vi "SCA-RT_Kubley-timing.vi"() -> ()   [LabVIEW 2016]
uses:
  controls/SCA states.ctl
  Common-Control/Gate Valve Readback.ctl
  controls/Vertical Rod states.ctl
  Common-Control/Horizontal Rod states.ctl
  Common-Control/GP307 cluster.ctl
  controls/SCA commands.ctl
  <vilib>/Platform/TimedLoop/XDataNode/timing_clust.ctl
  <vilib>/Platform/TimedLoop/XDataNode/nitl_modes.ctl
  <vilib>/Platform/TimedLoop/XDataNode/wakeup.ctl
  controls/Encoder bit cluster.ctl
  <vilib>/Analysis/baseanly.llb/Mean (DBL).vi
  <vilib>/Instr/_visa.llb/VISA Configure Serial Port (Instr).vi
  <vilib>/Motion/Express/_s/nimc.fb.straightLineMove.startStraightLineMove.axis.modeRelative.0.vi
  <vilib>/Platform/TimedLoop/XDataNode/loadnilvce.vi
  <vilib>/Motion/BlockNode/FB.NIMotion.xnode
  <vilib>/Platform/TimedLoop/XDataNode/XDataNode.xnode
  <vilib>/Platform/TimedLoop/XDataNode/XDNodeRunTimeDep.lvlib
  <vilib>/Analysis/NI_AALBase.lvlib
  <vilib>/NI_Real-Time Target Support.lvlib
panel:
  out "Immersion Lens I set":dbl
  out "Immersion Lens V Set":dbl
  out "Timeouts Update loop error":errorcluster
  out "SCA Command":T1
  out "Timeouts":T2
  out "Encoder loop error":errorcluster
  out "Convectron readback loop error":errorcluster
  out "HV Control loop error":errorcluster
  out "Rotate Wheel error":errorcluster
  out "Ion Source Vac Cluster":T3
  out "Bellows Vac Cluster":T3
  out "SCA-cRIO error":errorcluster
  in  "Rollover Sample":i8=54
  out "Insert Rod Status":T4
  out "Retract Rod Status":T4
  out "Sample Rod status":T5
  out "Wheel GV":T6
  out "Raw bits":bool[](array[boolean])
  out "Converted bits":bool[](array[boolean])
  out "Immersion Lens I read":dbl format="%0.2f"
  out "Immersion Lens V read":dbl format="%0.2f"
  out "SCA next state":T7
  out "Extractor I read":dbl
  out "Extractor V read":dbl
  out "Extractor V set":dbl
  out "Cathode V read":dbl
  out "Cathode I read":dbl
  out "Cathode V set":dbl
  in  "Execute Move":bool
  out "New Move":dbl
  out "Encoder Destination":dbl
  in  "Step Window Radius":i16=2
  out "In Range?":bool
  out "Window Limit 2":i16
  out "Window Limit 1":i16
  out "Encoder position":u16
  in  "clear error 3":bool
  in  "clear error 2":bool
  in  "clear error":bool
  out "action":string
  out "Vac Readback Loop error":errorcluster
  out "Sample Wheel Convectron":string
  out "Sample Rod UP sensor":bool
  out "Sample Rod DOWN sensor":bool
  out "done":bool
  out "Insert Rod IN sensor":bool
  out "Insert Rod OUT sensor":bool
  out "Retract Rod IN sensor":bool
  out "Retract Rod OUT sensor":bool
  out "Sensor loop error":errorcluster
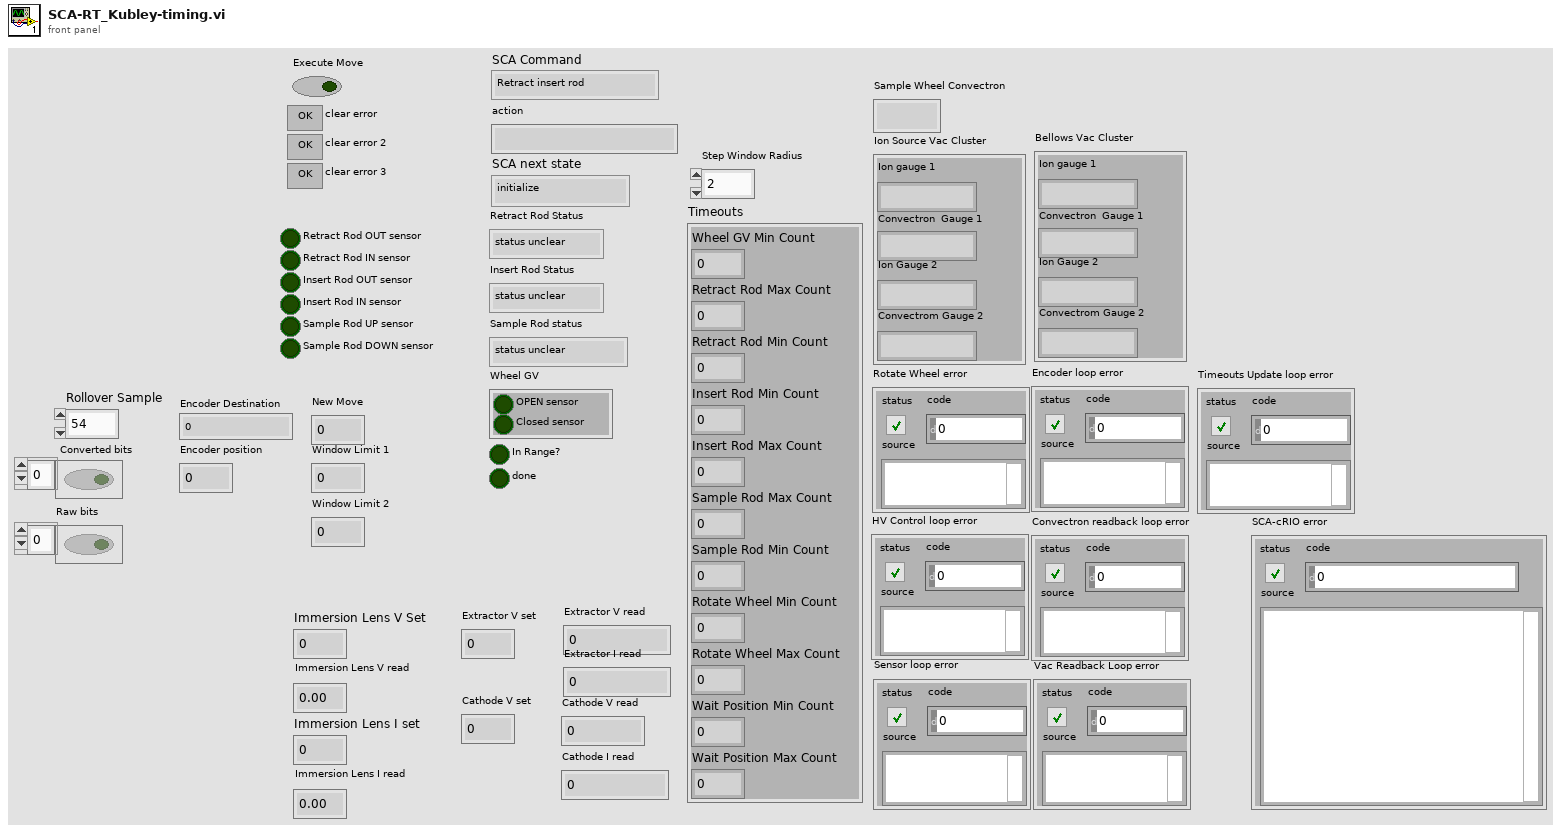
[diagram p1: front panel]
types:
  T1 = typedef "SCA commands.ctl" = enum16{"Retract insert rod", "Insert insert rod", "Retract retract rod", "Insert retract rod", "Retract sample rod", "Insert sample rod", "Open wheel GV", "Close wheel GV", "Open ion source GV", "Close ion source GV", "Pump out source", "Vent source", "Rotate wheel randomly", "Rotate wheel", "Start random sample change", "Start sample change"}
  T2 = cluster{"Wheel GV Min Count":i32, "Retract Rod Max Count":u32, "Retract Rod Min Count":u32, "Insert Rod Min Count":u32, "Insert Rod Max Count":u32, "Sample Rod Max Count":u32, "Sample Rod Min Count":u32, "Rotate Wheel Min Count":u32, "Rotate Wheel Max Count":u32, "Wait Position Min Count":u32, "Wait Position Max Count":u32}
  T3 = typedef "GP307 cluster.ctl" = cluster{"Ion gauge 1":string, "Convectron  Gauge 1 ":string, "Ion Gauge 2":string, "Convectrom Gauge 2":string}
  T4 = typedef "Horizontal Rod states.ctl" = enum16{"status unclear", "rod in", "rod out"}
  T5 = typedef "Vertical Rod states.ctl" = enum16{"status unclear", "rod down", "rod up"}
  T6 = typedef "Gate Valve Readback.ctl" = cluster{"OPEN sensor":bool, "Closed sensor":bool}
  T7 = typedef "SCA states.ctl" = enum16{"initialize", "wait", "change sample start", "change sample", "check position", "wait position", "rotate wheel", "sample change complete", "sample rod up", "sample rod down", "retract rod in", "retract rod out", "insert rod in", "insert rod out", "wheel GV open", "wheel GV close", "vent source", "pump source"}
  T8 = typedef "GV states.ctl" = enum16{"status unclear", "closed", "open"}
  T9 = typedef "XDNodeRunTimeDep.lvlib/timing_clust.ctl" = cluster{"Expected End [f-1]":u64, "Actual End [f-1]":u64, "Finished Late? [f-1]":bool, "Expected End [i-1]":u64, "Actual End [i-1]":u64, "Finished Late? [i-1]":bool, "Expected Start [i]":u64, "Actual Start [i]":u64, "Expected Start [f]":u64, "Actual Start [f]":u64, "Source Name":string, "Structure Name":string, "Period":i64, "Deadline":i64, "Offset":i64, "Start":i64, "Priority":i32, "Timeout":i32, "Mode":T10, "Wakeup Reason":T11, "Error":errorcluster, "Source Type":string, "Secondary Source Type":string, "Global End Time":u64, "Global Start Time":u64, "Frame Duration":u64, "Iteration Duration":u64, "Assigned CPU":i32, "I/O Scan Engine Mode":u32}
  T10 = typedef "XDNodeRunTimeDep.lvlib/nitl_modes.ctl" = enum32{"No Change", "Process missed periods, maintain original phase", "Discard missed periods, maintain original phase", "Process missed periods, ignore original phase", "Discard missed periods, ignore original phase"}
  T11 = typedef "XDNodeRunTimeDep.lvlib/wakeup.ctl" = enum32{"Normal", "Aborted", "Asynchronous wakeup", "Timing source error", "Timed loop error", "Timeout"}
  T12 = typedef "Encoder bit cluster.ctl" = cluster{"MSB":bool, "13th bit":bool, "12th bit":bool, "11th bit":bool, "10th bit":bool, "9th bit":bool, "8th bit":bool, "7th bit":bool, "6th bit":bool, "5th bit":bool, "4th bit":bool, "3rd bit":bool, "2nd bit":bool, "LSB":bool}
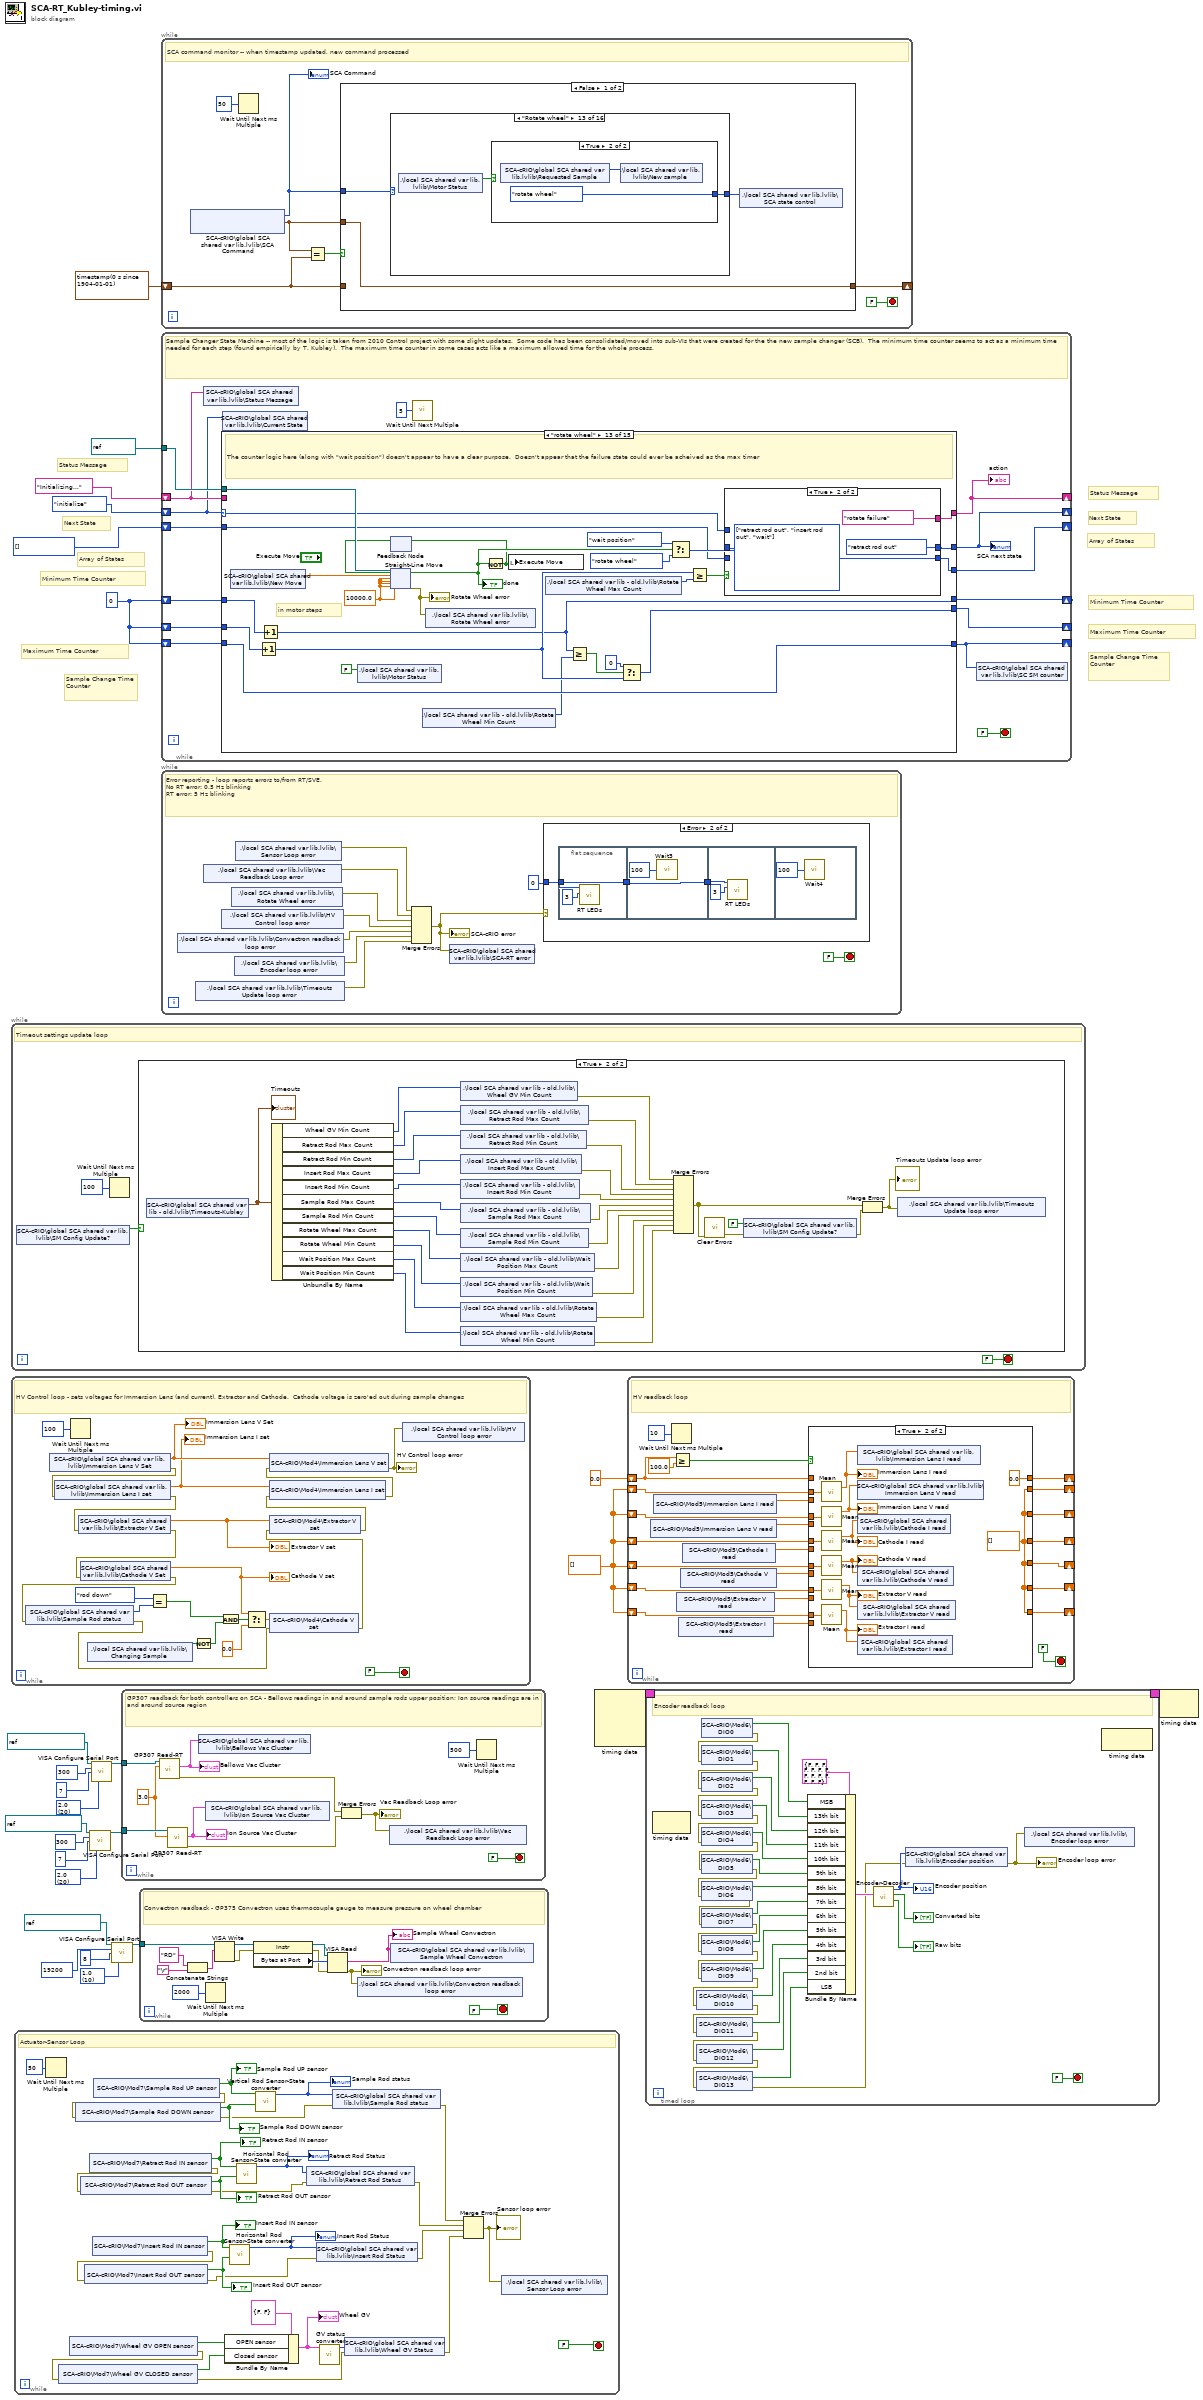
[diagram p0: block diagram]
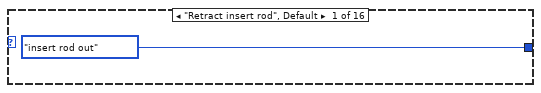
[diagram p2: hidden frame]
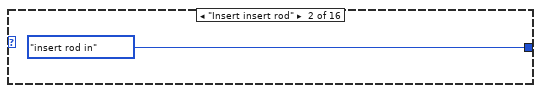
[diagram p3: hidden frame]
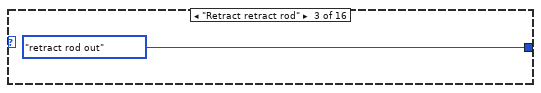
[diagram p4: hidden frame]
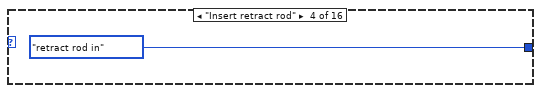
[diagram p5: hidden frame]
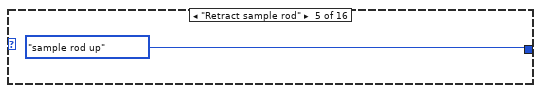
[diagram p6: hidden frame]
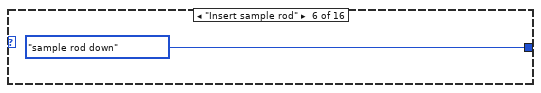
[diagram p7: hidden frame]
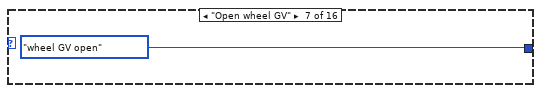
[diagram p8: hidden frame]
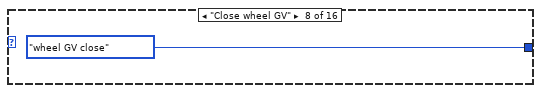
[diagram p9: hidden frame]
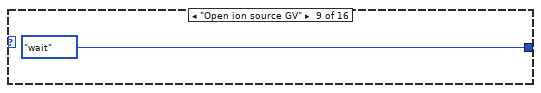
[diagram p10: hidden frame]
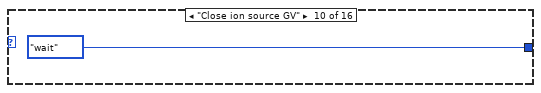
[diagram p11: hidden frame]
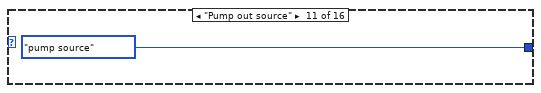
[diagram p12: hidden frame]
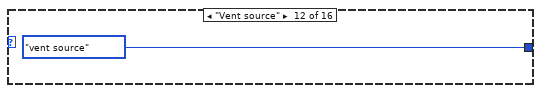
[diagram p13: hidden frame]
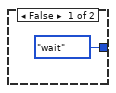
[diagram p14: hidden frame]
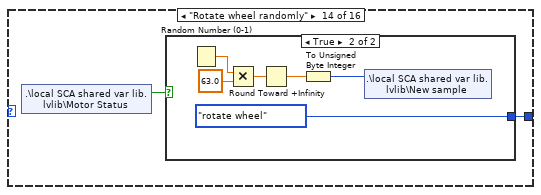
[diagram p15: hidden frame]
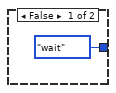
[diagram p16: hidden frame]
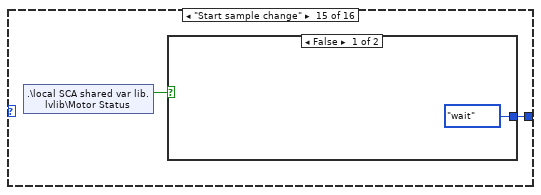
[diagram p17: hidden frame]
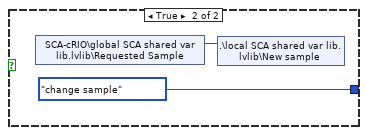
[diagram p18: hidden frame]
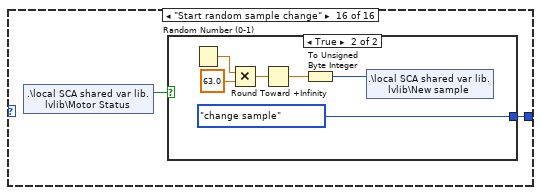
[diagram p19: hidden frame]
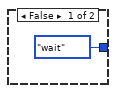
[diagram p20: hidden frame]
diagram:
  w3 = dbl[] []
  w20 = u16 20 items=["1.0"=10, "1.5"=15, "2.0"=20] ("stop bits (10: 1 bit)")
  w24 = u16 10 items=["1.0"=10, "1.5"=15, "2.0"=20] ("stop bits (10: 1 bit)")
  w14 = u16 20 items=["1.0"=10, "1.5"=15, "2.0"=20] ("stop bits (10: 1 bit)")
  w8 = u32 0
  w25 = T7[] [] items=["initialize", "wait", "change sample start", "change sample", "check position", "wait position", "rotate wheel", "sample change complete", "sample rod up", "sample rod down", "retract rod in", "retract rod out", "insert rod in", "insert rod out", "wheel GV open", "wheel GV close", "vent source", "pump source"]
  # "Status Message"
  # "Array of States"
  # "Next State"
  # "Sample Change Time Counter"
  # "Maximum Time Counter"
  # "Minimum Time Counter"
  # "Status Message"
  # "Array of States"
  # "Next State"
  # "Sample Change Time Counter"
  # "Maximum Time Counter"
  # "Minimum Time Counter"
  n1 = while {
    stop <- FALSE stop-if-true
    # "Timeout settings update loop"
    n2 = shared-variable "SCA-cRIO\\global SCA shared var lib.lvlib\\SM Config Update?"() -> (w28:bool)  [unwired: 1 in, 1 out]
    n3 = Wait Until Next ms Multiple(millisecond multiple=u32 100) -> ()  [unwired: 1 out]
    n4 = case shown="True" w28 {
      frame False {
      }
      frame True {
        n5 = shared-variable "SCA-cRIO\\global SCA shared var lib - old.lvlib\\Timeouts-Kubley"() -> (w55:T2)  [unwired: 1 in, 1 out]
        "Timeouts" <- w55
        n6 = Unbundle By Name(w55) -> ("Wheel GV Min Count"=w54:i32, "Retract Rod Max Count"=w53:u32, "Retract Rod Min Count"=w52:u32, "Insert Rod Max Count"=w51:u32, "Insert Rod Min Count"=w50:u32, "Sample Rod Max Count"=w49:u32, "Sample Rod Min Count"=w48:u32, "Rotate Wheel Max Count"=w47:u32, "Rotate Wheel Min Count"=w46:u32, "Wait Position Max Count"=w45:u32, "Wait Position Min Count"=w44:u32)
        n7 = shared-variable ".\\local SCA shared var lib - old.lvlib\\Wheel GV Min Count"(w54) -> (error out=w43:errorcluster)  [unwired: 1 in]
        n8 = shared-variable ".\\local SCA shared var lib - old.lvlib\\Retract Rod Max Count"(w53) -> (error out=w42:errorcluster)  [unwired: 1 in]
        n9 = shared-variable ".\\local SCA shared var lib - old.lvlib\\Retract Rod Min Count"(w52) -> (error out=w41:errorcluster)  [unwired: 1 in]
        n10 = shared-variable ".\\local SCA shared var lib - old.lvlib\\Insert Rod Max Count"(w51) -> (error out=w40:errorcluster)  [unwired: 1 in]
        n11 = shared-variable ".\\local SCA shared var lib - old.lvlib\\Insert Rod Min Count"(w50) -> (error out=w39:errorcluster)  [unwired: 1 in]
        n12 = shared-variable ".\\local SCA shared var lib - old.lvlib\\Sample Rod Max Count"(w49) -> (error out=w38:errorcluster)  [unwired: 1 in]
        n13 = shared-variable ".\\local SCA shared var lib - old.lvlib\\Sample Rod Min Count"(w48) -> (error out=w37:errorcluster)  [unwired: 1 in]
        n14 = shared-variable ".\\local SCA shared var lib - old.lvlib\\Wait Position Max Count"(w47) -> (error out=w36:errorcluster)  [unwired: 1 in]
        n15 = shared-variable ".\\local SCA shared var lib - old.lvlib\\Wait Position Min Count"(w46) -> (error out=w35:errorcluster)  [unwired: 1 in]
        n16 = shared-variable ".\\local SCA shared var lib - old.lvlib\\Rotate Wheel Max Count"(w45) -> (error out=w34:errorcluster)  [unwired: 1 in]
        n17 = shared-variable ".\\local SCA shared var lib - old.lvlib\\Rotate Wheel Min Count"(w44) -> (error out=w33:errorcluster)  [unwired: 1 in]
        n18 = Merge Errors(w43, w42, w41, w40, w39, w38, w37, w36, w35, w34, w33) -> (w31:errorcluster)
        n19 = call <vilib>:"Clear Errors.vi"("error in (no error)"=w31) -> ("error out"=w32:errorcluster)  [unwired: 5 in, 1 out]
        n20 = shared-variable "SCA-cRIO\\global SCA shared var lib.lvlib\\SM Config Update?"(FALSE ("SM Config Update?"), error in=w32) -> (error out=w30:errorcluster)
        n21 = Merge Errors(w31, w30) -> (w29:errorcluster)
        "Timeouts Update loop error" <- w29
        n22 = shared-variable ".\\local SCA shared var lib.lvlib\\Timeouts Update loop error"(w29) -> ()  [unwired: 1 in, 1 out]
      }
    }
  }
  n23 = while {
    stop <- FALSE stop-if-true
    # "HV Control loop - sets voltages for Immersion Lens (and current), Extractor and Cathode.  Cathode voltage is zero'ed out during sample changes"
    n24 = shared-variable "SCA-cRIO\\global SCA shared var lib.lvlib\\Immersion Lens V Set"() -> (w71:dbl, error out=w69:errorcluster)  [unwired: 1 in]
    "Immersion Lens V Set" <- w71
    n25 = shared-variable "SCA-cRIO\\global SCA shared var lib.lvlib\\Immersion Lens I set"(error in=w69) -> (w70:dbl, error out=w68:errorcluster)
    "Immersion Lens I set" <- w70
    n26 = Wait Until Next ms Multiple(millisecond multiple=u32 100) -> ()  [unwired: 1 out]
    n27 = shared-variable "SCA-cRIO\\global SCA shared var lib.lvlib\\Extractor V Set"(error in=w68) -> (w77:dbl, error out=w67:errorcluster)
    "Extractor V set" <- w77
    n28 = shared-variable "SCA-cRIO\\global SCA shared var lib.lvlib\\Cathode V Set"(error in=w67) -> (w74:dbl, error out=w66:errorcluster)
    "Cathode V set" <- w74
    n29 = shared-variable "SCA-cRIO\\global SCA shared var lib.lvlib\\Sample Rod status"(error in=w66) -> (w60:T5, error out=w58:errorcluster)
    n30 = shared-variable ".\\local SCA shared var lib.lvlib\\Changing Sample"() -> (w76:bool)  [unwired: 1 in, 1 out]
    n31 = Equal?(x=Vertical_Rod_states."rod down", y=w60) -> (x = y?=w61:bool)
    n32 = Not(x=w76) -> (.not. x?=w57:bool)
    n33 = And(x=w61, y=w57) -> (x .and. y?=w75:bool)
    n34 = Select(t=w74, s=w75, f=0.0) -> (s? t:f=w72:dbl)
    n35 = shared-variable "SCA-cRIO\\Mod4\\Cathode V set"(w72, error in=w58) -> (error out=w63:errorcluster)
    n36 = shared-variable "SCA-cRIO\\Mod4\\Extractor V set"(w77, error in=w63) -> (error out=w64:errorcluster)
    n37 = shared-variable "SCA-cRIO\\Mod4\\Immersion Lens I set"(w70, error in=w64) -> (error out=w65:errorcluster)
    n38 = shared-variable "SCA-cRIO\\Mod4\\Immersion Lens V set"(w71, error in=w65) -> (error out=w62:errorcluster)
    "HV Control loop error" <- w62
    n39 = shared-variable ".\\local SCA shared var lib.lvlib\\HV Control loop error"(w62) -> ()  [unwired: 1 in, 1 out]
  }
  n40 = while {
    stop <- FALSE ("stop") stop-if-true
    # "Actuator-Sensor Loop"
    n41 = Wait Until Next ms Multiple(millisecond multiple=u32 50) -> ()  [unwired: 1 out]
    n42 = shared-variable "SCA-cRIO\\Mod7\\Wheel GV OPEN sensor"() -> (w103:bool, error out=w89:errorcluster)  [unwired: 1 in]
    n43 = shared-variable "SCA-cRIO\\Mod7\\Wheel GV CLOSED sensor"(error in=w89) -> (w104:bool, error out=w88:errorcluster)
    n44 = shared-variable "SCA-cRIO\\Mod7\\Retract Rod IN sensor"() -> (w98:bool, error out=w91:errorcluster)  [unwired: 1 in]
    "Retract Rod IN sensor" <- w98
    n45 = shared-variable "SCA-cRIO\\Mod7\\Retract Rod OUT sensor"(error in=w91) -> (w97:bool, error out=w85:errorcluster)
    "Retract Rod OUT sensor" <- w97
    n46 = shared-variable "SCA-cRIO\\Mod7\\Insert Rod IN sensor"() -> (w96:bool, error out=w90:errorcluster)  [unwired: 1 in]
    "Insert Rod IN sensor" <- w96
    n47 = shared-variable "SCA-cRIO\\Mod7\\Insert Rod OUT sensor"(error in=w90) -> (w95:bool, error out=w87:errorcluster)
    "Insert Rod OUT sensor" <- w95
    n48 = shared-variable "SCA-cRIO\\Mod7\\Sample Rod UP sensor"() -> (w101:bool, error out=w92:errorcluster)  [unwired: 1 in]
    "Sample Rod UP sensor" <- w101
    n49 = shared-variable "SCA-cRIO\\Mod7\\Sample Rod DOWN sensor"(error in=w92) -> (w100:bool, error out=w86:errorcluster)
    "Sample Rod DOWN sensor" <- w100
    n50 = Bundle By Name(cluster=T6 {"OPEN sensor"=FALSE, "Closed sensor"=FALSE} ("Gate Valve"), "OPEN sensor"=w103, "Closed sensor"=w104) -> (w106:T6)
    "Wheel GV" <- w106
    n51 = call "Horizontal Rod Sensor-State converter.vi"("IN Sensor"=w96, "OUT Sensor"=w95) -> ("Status"=w94:T4)  [unwired: 8 in]
    "Insert Rod Status" <- w94
    n52 = call "Horizontal Rod Sensor-State converter.vi"("IN Sensor"=w98, "OUT Sensor"=w97) -> ("Status"=w93:T4)  [unwired: 8 in]
    "Retract Rod Status" <- w93
    n53 = call "Vertical Rod Sensor-State converter.vi"("UP Sensor"=w101, "DOWN Sensor"=w100) -> ("Status"=w99:T5)  [unwired: 8 in]
    "Sample Rod status" <- w99
    n54 = shared-variable "SCA-cRIO\\global SCA shared var lib.lvlib\\Retract Rod Status"(w93, error in=w85) -> (error out=w82:errorcluster)
    n55 = shared-variable "SCA-cRIO\\global SCA shared var lib.lvlib\\Insert Rod Status"(w94, error in=w87) -> (error out=w81:errorcluster)
    n56 = call "GV status converter.vi"("Gate Valve"=w106) -> ("GV Status"=w102:T8)  [unwired: 10 in]
    n57 = shared-variable "SCA-cRIO\\global SCA shared var lib.lvlib\\Sample Rod status"(w99, error in=w86) -> (error out=w83:errorcluster)
    n58 = shared-variable "SCA-cRIO\\global SCA shared var lib.lvlib\\Wheel GV Status"(w102, error in=w88) -> (error out=w80:errorcluster)
    n59 = Merge Errors(w83, w82, w81, w80) -> (w84:errorcluster)
    "Sensor loop error" <- w84
    n60 = shared-variable ".\\local SCA shared var lib.lvlib\\Sensor Loop error"(w84) -> ()  [unwired: 1 in, 1 out]
  }
  n61 = call-poly "VISA Configure Serial Port"("VISA resource name"=refnum<visa-resource-name> "ASRL6::INSTR", "baud rate (9600)"=u32 300, "data bits (8)"=u16 7, "stop bits (10: 1 bit)"=w14) -> ("VISA resource name out"=w15:refnum<visa-resource-name>)  [unwired: 10 in, 1 out]
  n62 = call-poly "VISA Configure Serial Port"("VISA resource name"=refnum<visa-resource-name> "ASRL8::INSTR", "baud rate (9600)"=u32 300, "data bits (8)"=u16 7, "stop bits (10: 1 bit)"=w20) -> ("VISA resource name out"=w21:refnum<visa-resource-name>)  [unwired: 10 in, 1 out]
  n63 = call-poly "VISA Configure Serial Port"("VISA resource name"=refnum<visa-resource-name> "ASRL7::INSTR", "baud rate (9600)"=u32 19200, "data bits (8)"=u16 8, "stop bits (10: 1 bit)"=w24) -> ("VISA resource name out"=w10:refnum<visa-resource-name>)  [unwired: 10 in, 1 out]
  n64 = while {
    tunnel: w15 -> [w112]
    tunnel: w21 -> [w115]
    stop <- FALSE ("stop 4") stop-if-true
    w111 = 3.0 ("Delay Time (s)")
    # "GP307 readback for both controllers on SCA - Bellows readings in and around sample rods upper position; Ion source readings are in and around source region"
    n65 = call "GP307 Read-RT.vi"("Delay Time (s)"=w111, "VISA Refnum in"=w115) -> ("error out"=w113:errorcluster, "GP307 output"=w114:T3)  [unwired: 7 in, 1 out]
    "Bellows Vac Cluster" <- w114
    n66 = call "GP307 Read-RT.vi"("Delay Time (s)"=w111, "VISA Refnum in"=w112) -> ("error out"=w109:errorcluster, "GP307 output"=w110:T3)  [unwired: 7 in, 1 out]
    "Ion Source Vac Cluster" <- w110
    n67 = shared-variable "SCA-cRIO\\global SCA shared var lib.lvlib\\Bellows Vac Cluster"(w114) -> ()  [unwired: 1 in, 1 out]
    n68 = shared-variable "SCA-cRIO\\global SCA shared var lib.lvlib\\Ion Source Vac Cluster"(w110) -> ()  [unwired: 1 in, 1 out]
    n69 = Merge Errors(w113, w109) -> (w116:errorcluster)
    "Vac Readback Loop error" <- w116
    n70 = shared-variable ".\\local SCA shared var lib.lvlib\\Vac Readback Loop error"(w116) -> ()  [unwired: 1 in, 1 out]
    n71 = Wait Until Next ms Multiple(millisecond multiple=u32 500) -> ()  [unwired: 1 out]
  }
  n72 = while {
    tunnel: w10 -> [w124]
    stop <- FALSE ("stop 3") stop-if-true
    # "Convectron readback - GP375 Convectron uses thermocouple gauge to measure pressure on wheel chamber"
    n73 = Concatenate Strings("RD" ("write buffer 2"), "\r") -> (w131:string)
    n74 = Wait Until Next ms Multiple(millisecond multiple=u32 2000) -> ()  [unwired: 1 out]
    n75 = VISA Write(VISA resource name=w124, write buffer=w131) -> (VISA resource name out=w125:refnum<visa-resource-name>, error out=w121:errorcluster)  [unwired: 1 in, 1 out]
    n76 = property class="Instr"(reference=w125, error in=w121) -> (reference out=w126:refnum<visa-resource-name>, error out=w120:errorcluster, "Bytes at Port"=w127:u32)
    n77 = VISA Read(VISA resource name=w126, byte count=w127, error in (no error)=w120) -> (read buffer=w122:string, error out=w119:errorcluster)  [unwired: 2 out]
    "Sample Wheel Convectron" <- w122
    "Convectron readback loop error" <- w119
    n78 = shared-variable ".\\local SCA shared var lib.lvlib\\Convectron readback loop error"(w119) -> ()  [unwired: 1 in, 1 out]
    n79 = shared-variable "SCA-cRIO\\global SCA shared var lib.lvlib\\Sample Wheel Convectron"(w122) -> ()  [unwired: 1 in, 1 out]
  }
  n80 = while {
    shift-right: [w144] -> _
    shift-left: SCA_states."initialize" ("SC2 state") -> [w134]
    shift-right: [w133] -> _
    shift-left: w25 -> [w143]
    shift-right: [w141] -> _
    shift-left: w8 -> [w142]
    shift-right: [w140] -> _
    shift-left: "Initializing..." -> [w135]
    shift-right: [w138] -> _
    shift-left: w8 -> [w139]
    shift-right: [w136] -> _
    shift-left: w8 -> [w137]
    tunnel: refnum<k21> "Axis 1" ("resource") -> [w145]
    stop <- FALSE ("stop 2") stop-if-true
    # "Sample Changer State Machine -- most of the logic is taken from 2010 Control project with some slight updates.  Some code has been consolidated/moved into sub-VIs that were created for the the new sample changer (SCB).  The minimum time counter seems to act as a minimum time needed for each step (found empirically by T. Kubley).  The maximum time counter in some cases acts like a maximum allowed time for the whole process."
    n81 = shared-variable "SCA-cRIO\\global SCA shared var lib.lvlib\\Status Message"(w135) -> ()  [unwired: 1 in, 1 out]
    n82 = case shown="\"rotate wheel\"" w134 {
      selector: w134 -> [_ _ _ _ w219 w237 w260 w294 w328 w362 w396 w430 w466 w521 w551]
      tunnel: w145 -> [_ _ _ _ _ _ _ _ _ _ _ _ w481 _ _]
      tunnel: [SCA_states."wait" ("SC2 state") w170 w200 w210 w224 w243 w268 w302 w336 w370 w404 w438 w475 w522 w561] -> w144
      tunnel: w143 -> [w160 _ w192 w202 w220 w238 w261 w295 w329 w363 w397 w431 w467 w520 w550]
      tunnel: w142 -> [w163 _ _ _ w227 w246 w274 w308 w342 w376 w410 w444 w479 w532 w556]
      tunnel: [w163 w173 w195 w205 w226 w245 w254 w288 w323 w357 w391 w425 w462 w533 w556] -> w141
      tunnel: [w160 w171 w192 w202 w220 w238 w263 w297 w331 w365 w399 w433 w476 w529 w550] -> w133
      tunnel: w135 -> [w161 w176 w198 w208 _ _ _ _ _ _ _ _ _ _ _]
      tunnel: [w161 w175 w197 w207 w223 w242 w270 w304 w338 w372 w406 w440 w474 w528 w560] -> w140
      tunnel: w139 -> [w164 _ _ _ w225 w244 w267 w301 w335 w369 w403 w437 w477 w530 _]
      tunnel: [w164 w173 w195 w205 w212 w241 w265 w299 w333 w367 w401 w435 w470 w524 u32 0 ("t")] -> w138
      tunnel: w137 -> [w165 _ _ _ w222 w240 w264 w298 w332 w366 w400 w434 w461 w517 w559]
      tunnel: [w165 w173 w195 w205 w222 w240 w264 w298 w332 w366 w400 w434 w461 w517 w559] -> w136
      frame "initialize" {
        n83 = shared-variable ".\\local SCA shared var lib.lvlib\\Motor Status"(TRUE ("Motor Status")) -> ()  [unwired: 1 in, 1 out]
        n84 = shared-variable ".\\local SCA shared var lib.lvlib\\Changing Sample"(FALSE ("Changing Sample")) -> ()  [unwired: 1 in, 1 out]
        n85 = shared-variable "SCA-cRIO\\global SCA shared var lib - old.lvlib\\Start Sample Change"(FALSE ("start sample change")) -> (error out=w168:errorcluster)  [unwired: 1 in]
        n86 = shared-variable ".\\local SCA shared var lib - old.lvlib\\Rotate Wheel Max Count"(u32 800 ("Rotate Wheel Max Count")) -> ()  [unwired: 1 in, 1 out]
        n87 = shared-variable ".\\local SCA shared var lib - old.lvlib\\Wait Position Min Count"(u32 8000 ("y")) -> ()  [unwired: 1 in, 1 out]
        n88 = shared-variable ".\\local SCA shared var lib - old.lvlib\\Wait Position Max Count"(u32 1500 ("y")) -> ()  [unwired: 1 in, 1 out]
        n89 = shared-variable ".\\local SCA shared var lib - old.lvlib\\Rotate Wheel Min Count"(u32 350 ("Rotate Wheel Min Count")) -> ()  [unwired: 1 in, 1 out]
        n90 = shared-variable "SCA-cRIO\\global SCA shared var lib - old.lvlib\\change sample start end"(FALSE ("change sample start end"), error in=w168) -> ()  [unwired: 1 out]
        n91 = shared-variable ".\\local SCA shared var lib - old.lvlib\\Insert Rod Min Count"(u32 30 ("y")) -> ()  [unwired: 1 in, 1 out]
        n92 = shared-variable ".\\local SCA shared var lib - old.lvlib\\Insert Rod Max Count"(u32 500 ("y")) -> ()  [unwired: 1 in, 1 out]
        n93 = shared-variable ".\\local SCA shared var lib - old.lvlib\\Wheel GV Min Count"(70 ("Wheel GV Min Time")) -> ()  [unwired: 1 in, 1 out]
        n94 = shared-variable ".\\local SCA shared var lib - old.lvlib\\Sample Rod Min Count"(u32 10 ("y")) -> ()  [unwired: 1 in, 1 out]
        n95 = shared-variable ".\\local SCA shared var lib - old.lvlib\\Sample Rod Max Count"(u32 1000 ("y")) -> ()  [unwired: 1 in, 1 out]
        n96 = shared-variable ".\\local SCA shared var lib - old.lvlib\\Retract Rod Max Count"(u32 200 ("y")) -> ()  [unwired: 1 in, 1 out]
        n97 = shared-variable ".\\local SCA shared var lib - old.lvlib\\Retract Rod Min Count"(u32 30 ("y")) -> ()  [unwired: 1 in, 1 out]
      }
      frame "wait", Default {
        w173 = u32 0
        n98 = shared-variable ".\\local SCA shared var lib.lvlib\\SCA state control"() -> (w169:T7)  [unwired: 1 in, 1 out]
        n99 = case shown="\"change sample\"" w169 {
          tunnel: [w178 w179 w180 w181 w182 w183 w184 w185 w186 w187 w188 w189 w190] -> w171
          frame "wheel GV close" {
            w178 = T7[] [enum."wheel GV close", enum."wait"] items=["initialize", "wait", "change sample start", "change sample", "check position", "wait position", "rotate wheel", "sample change complete", "sample rod up", "sample rod down", "retract rod in", "retract rod out", "insert rod in", "insert rod out", "wheel GV open", "wheel GV close", "vent source", "pump source"]
          }
          frame "wheel GV open" {
            w179 = T7[] [enum."wheel GV open", enum."wait"] items=["initialize", "wait", "change sample start", "change sample", "check position", "wait position", "rotate wheel", "sample change complete", "sample rod up", "sample rod down", "retract rod in", "retract rod out", "insert rod in", "insert rod out", "wheel GV open", "wheel GV close", "vent source", "pump source"]
          }
          frame "sample rod up" {
            w180 = T7[] [enum."sample rod up", enum."wait"] items=["initialize", "wait", "change sample start", "change sample", "check position", "wait position", "rotate wheel", "sample change complete", "sample rod up", "sample rod down", "retract rod in", "retract rod out", "insert rod in", "insert rod out", "wheel GV open", "wheel GV close", "vent source", "pump source"]
          }
          frame "sample rod down" {
            w181 = T7[] [enum."sample rod down", enum."wait"] items=["initialize", "wait", "change sample start", "change sample", "check position", "wait position", "rotate wheel", "sample change complete", "sample rod up", "sample rod down", "retract rod in", "retract rod out", "insert rod in", "insert rod out", "wheel GV open", "wheel GV close", "vent source", "pump source"]
          }
          frame "retract rod in" {
            w182 = T7[] [enum."retract rod in", enum."wait"] items=["initialize", "wait", "change sample start", "change sample", "check position", "wait position", "rotate wheel", "sample change complete", "sample rod up", "sample rod down", "retract rod in", "retract rod out", "insert rod in", "insert rod out", "wheel GV open", "wheel GV close", "vent source", "pump source"]
          }
          frame "retract rod out" {
            w183 = T7[] [enum."retract rod out", enum."wait"] items=["initialize", "wait", "change sample start", "change sample", "check position", "wait position", "rotate wheel", "sample change complete", "sample rod up", "sample rod down", "retract rod in", "retract rod out", "insert rod in", "insert rod out", "wheel GV open", "wheel GV close", "vent source", "pump source"]
          }
          frame "insert rod in" {
            w184 = T7[] [enum."insert rod in", enum."wait"] items=["initialize", "wait", "change sample start", "change sample", "check position", "wait position", "rotate wheel", "sample change complete", "sample rod up", "sample rod down", "retract rod in", "retract rod out", "insert rod in", "insert rod out", "wheel GV open", "wheel GV close", "vent source", "pump source"]
          }
          frame "insert rod out" {
            w185 = T7[] [enum."insert rod out", enum."wait"] items=["initialize", "wait", "change sample start", "change sample", "check position", "wait position", "rotate wheel", "sample change complete", "sample rod up", "sample rod down", "retract rod in", "retract rod out", "insert rod in", "insert rod out", "wheel GV open", "wheel GV close", "vent source", "pump source"]
          }
          frame "rotate wheel" {
            w186 = T7[] [enum."check position", enum."wait"] items=["initialize", "wait", "change sample start", "change sample", "check position", "wait position", "rotate wheel", "sample change complete", "sample rod up", "sample rod down", "retract rod in", "retract rod out", "insert rod in", "insert rod out", "wheel GV open", "wheel GV close", "vent source", "pump source"]
          }
          frame "change sample" {
            w187 = T7[] [enum."change sample start", enum."sample rod up", enum."retract rod in", enum."retract rod out", enum."check position", enum."insert rod in", enum."insert rod out", enum."sample rod down", enum."sample change complete", enum."wait"] items=["initialize", "wait", "change sample start", "change sample", "check position", "wait position", "rotate wheel", "sample change complete", "sample rod up", "sample rod down", "retract rod in", "retract rod out", "insert rod in", "insert rod out", "wheel GV open", "wheel GV close", "vent source", "pump source"]
          }
          frame "vent source" {
            w188 = T7[] [enum."sample rod up", enum."retract rod in", enum."retract rod out", enum."insert rod out", enum."wheel GV close", enum."wait"] items=["initialize", "wait", "change sample start", "change sample", "check position", "wait position", "rotate wheel", "sample change complete", "sample rod up", "sample rod down", "retract rod in", "retract rod out", "insert rod in", "insert rod out", "wheel GV open", "wheel GV close", "vent source", "pump source"]
          }
          frame "pump source" {
            w189 = T7[] [enum."wheel GV open", enum."sample rod up", enum."check position", enum."insert rod in", enum."insert rod out", enum."sample rod down", enum."wait"] items=["initialize", "wait", "change sample start", "change sample", "check position", "wait position", "rotate wheel", "sample change complete", "sample rod up", "sample rod down", "retract rod in", "retract rod out", "insert rod in", "insert rod out", "wheel GV open", "wheel GV close", "vent source", "pump source"]
          }
          frame "wait", Default {
            w190 = T7[] [enum."wait"] items=["initialize", "wait", "change sample start", "change sample", "check position", "wait position", "rotate wheel", "sample change complete", "sample rod up", "sample rod down", "retract rod in", "retract rod out", "insert rod in", "insert rod out", "wheel GV open", "wheel GV close", "vent source", "pump source"]
          }
        }
        n100 = Select(t="Ready", s="clear error", f=w176) -> (s? t:f=w175:string)
        n101 = Index Array(array=w171, index=0) -> (element=w170:T7)
      }
      frame "change sample start" {
        w195 = u32 0
        n102 = Index Array(array=w192, index=1) -> (element=w200:T7)
        n103 = shared-variable "SCA-cRIO\\global SCA shared var lib - old.lvlib\\change sample start end"(FALSE ("change sample start end")) -> ()  [unwired: 1 in, 1 out]
        n104 = shared-variable ".\\local SCA shared var lib.lvlib\\Changing Sample"(TRUE ("Changing Sample")) -> ()  [unwired: 1 in, 1 out]
        n105 = Select(t="Ready", s="clear error 2", f=w198) -> (s? t:f=w197:string)
      }
      frame "sample change complete" {
        w205 = u32 0
        n106 = shared-variable "SCA-cRIO\\global SCA shared var lib - old.lvlib\\change sample start end"(TRUE ("change sample start end")) -> ()  [unwired: 1 in, 1 out]
        n107 = shared-variable ".\\local SCA shared var lib.lvlib\\Changing Sample"(FALSE ("Changing Sample")) -> ()  [unwired: 1 in, 1 out]
        n108 = Array Size(array=w202) -> (size(s)=w203:i32)
        n109 = Index Array(array=w202, index=w203) -> (element=w210:T7)
        n110 = Select(t="Ready", s="clear error 3", f=w208) -> (s? t:f=w207:string)
      }
      frame "wheel GV open" {
        n111 = call "Modify array of SCA states.vi"("Current State"=w219, "Array of states to process"=w220) -> ("Next State"=w221:T7)  [unwired: 7 in, 1 out]
        n112 = shared-variable "SCA-cRIO\\Mod8\\Wheel GV Actuator"(TRUE ("sc gate valve")) -> (error out=w217:errorcluster)  [unwired: 1 in]
        n113 = shared-variable "SCA-cRIO\\global SCA shared var lib.lvlib\\Wheel GV Status"(error in=w217) -> (w216:enum16{"status unclear", "closed", "open"})  [unwired: 1 out]
        n114 = shared-variable ".\\local SCA shared var lib - old.lvlib\\Wheel GV Min Count"() -> (w211:i32)  [unwired: 1 in, 1 out]
        n115 = Equal?(x=enum16{"status unclear", "closed", "open"}."open", y=w216) -> (x = y?=w214:bool)
        n116 = Select(t=w227, s=w214, f=u32 0) -> (s? t:f=w230:u32)
        n117 = Increment(x=w230) -> (x+1=w226:u32)
        n118 = Greater Or Equal?(x=w226, y=w211) -> (x >= y?=w228:bool)
        n119 = Select(t=w221, s=w228, f=w219) -> (s? t:f=w224:T7)
        n120 = Increment(x=w225) -> (x+1=w212:u32)
        n121 = Format Into String(format string="%s", w219) -> (resulting string=w223:string)  [unwired: 2 in, 1 out]
      }
      frame "wheel GV close" {
        n122 = call "Modify array of SCA states.vi"("Current State"=w237, "Array of states to process"=w238) -> ("Next State"=w239:T7)  [unwired: 7 in, 1 out]
        n123 = shared-variable "SCA-cRIO\\Mod8\\Wheel GV Actuator"(FALSE ("sc gate valve")) -> (error out=w235:errorcluster)  [unwired: 1 in]
        n124 = shared-variable "SCA-cRIO\\global SCA shared var lib.lvlib\\Wheel GV Status"(error in=w235) -> (w234:enum16{"status unclear", "closed", "open"})  [unwired: 1 out]
        n125 = shared-variable ".\\local SCA shared var lib - old.lvlib\\Wheel GV Min Count"() -> (w250:i32)  [unwired: 1 in, 1 out]
        n126 = Equal?(x=enum16{"status unclear", "closed", "open"}."closed", y=w234) -> (x = y?=w232:bool)
        n127 = Select(t=w246, s=w232, f=u32 0) -> (s? t:f=w249:u32)
        n128 = Increment(x=w249) -> (x+1=w245:u32)
        n129 = Greater Or Equal?(x=w245, y=w250) -> (x >= y?=w247:bool)
        n130 = Select(t=w239, s=w247, f=w237) -> (s? t:f=w243:T7)
        n131 = Increment(x=w244) -> (x+1=w241:u32)
        n132 = Format Into String(format string="%s", w237) -> (resulting string=w242:string)  [unwired: 2 in, 1 out]
      }
      frame "sample rod up" {
        n133 = Increment(x=w267) -> (x+1=w253:u32)
        n134 = shared-variable "SCA-cRIO\\Mod8\\Sample Rod Actuator"(FALSE ("Sample Rod Actuator")) -> (error out=w258:errorcluster)  [unwired: 1 in]
        n135 = shared-variable ".\\local SCA shared var lib - old.lvlib\\Sample Rod Max Count"() -> (w252:u32)  [unwired: 1 in, 1 out]
        n136 = call "Modify array of SCA states.vi"("Current State"=w260, "Array of states to process"=w261) -> ("Next State"=w262:T7)  [unwired: 7 in, 1 out]
        n137 = shared-variable "SCA-cRIO\\global SCA shared var lib.lvlib\\Sample Rod status"(error in=w258) -> (w257:T5)  [unwired: 1 out]
        n138 = Greater Or Equal?(x=w253, y=w252) -> (x >= y?=w266:bool)
        n139 = shared-variable ".\\local SCA shared var lib - old.lvlib\\Sample Rod Min Count"() -> (w251:u32)  [unwired: 1 in, 1 out]
        n140 = Equal?(x=w257, y=Vertical_Rod_states."rod up") -> (x = y?=w255:bool)
        n141 = Select(t=w274, s=w255, f=u32 0) -> (s? t:f=w272:u32)
        n142 = Increment(x=w272) -> (x+1=w254:u32)
        n143 = Greater Or Equal?(x=w254, y=w251) -> (x >= y?=w273:bool)
        n144 = Select(t=w262, s=w273, f=w260) -> (s? t:f=w269:T7)
        n145 = case shown="False" w266 {
          tunnel: [w280 u32 0] -> w265
          tunnel: [w278 w281] -> w263
          tunnel: [w279 SCA_states."wait" ("SC2 state")] -> w268
          tunnel: w253 -> [w280 _]
          tunnel: w260 -> [w276 _]
          tunnel: [w275 "sample rod failure"] -> w270
          tunnel: w269 -> [w279 _]
          tunnel: w261 -> [w278 _]
          frame False {
            n146 = Format Into String(format string="%s", w276) -> (resulting string=w275:string)  [unwired: 2 in, 1 out]
          }
          frame True {
            w281 = T7[] [enum."wait", enum."insert rod out", enum."wait"] items=["initialize", "wait", "change sample start", "change sample", "check position", "wait position", "rotate wheel", "sample change complete", "sample rod up", "sample rod down", "retract rod in", "retract rod out", "insert rod in", "insert rod out", "wheel GV open", "wheel GV close", "vent source", "pump source"]
          }
        }
      }
      frame "sample rod down" {
        n147 = Increment(x=w301) -> (x+1=w287:u32)
        n148 = shared-variable "SCA-cRIO\\Mod8\\Sample Rod Actuator"(TRUE ("Sample Rod Actuator")) -> (error out=w292:errorcluster)  [unwired: 1 in]
        n149 = shared-variable ".\\local SCA shared var lib - old.lvlib\\Sample Rod Max Count"() -> (w285:u32)  [unwired: 1 in, 1 out]
        n150 = call "Modify array of SCA states.vi"("Current State"=w294, "Array of states to process"=w295) -> ("Next State"=w296:T7)  [unwired: 7 in, 1 out]
        n151 = shared-variable "SCA-cRIO\\global SCA shared var lib.lvlib\\Sample Rod status"(error in=w292) -> (w291:T5)  [unwired: 1 out]
        n152 = Greater Or Equal?(x=w287, y=w285) -> (x >= y?=w300:bool)
        n153 = shared-variable ".\\local SCA shared var lib - old.lvlib\\Sample Rod Min Count"() -> (w286:u32)  [unwired: 1 in, 1 out]
        n154 = Equal?(x=w291, y=Vertical_Rod_states."rod down") -> (x = y?=w289:bool)
        n155 = Select(t=w308, s=w289, f=u32 0) -> (s? t:f=w306:u32)
        n156 = Increment(x=w306) -> (x+1=w288:u32)
        n157 = Greater Or Equal?(x=w288, y=w286) -> (x >= y?=w307:bool)
        n158 = Select(t=w296, s=w307, f=w294) -> (s? t:f=w303:T7)
        n159 = case shown="True" w300 {
          tunnel: [w314 u32 0] -> w299
          tunnel: [w312 w315] -> w297
          tunnel: [w313 SCA_states."wait" ("SC2 state")] -> w302
          tunnel: w287 -> [w314 _]
          tunnel: w294 -> [w310 _]
          tunnel: [w309 "sample rod failure"] -> w304
          tunnel: w303 -> [w313 _]
          tunnel: w295 -> [w312 _]
          frame False {
            n160 = Format Into String(format string="%s", w310) -> (resulting string=w309:string)  [unwired: 2 in, 1 out]
          }
          frame True {
            w315 = T7[] [enum."wait", enum."insert rod out", enum."wait"] items=["initialize", "wait", "change sample start", "change sample", "check position", "wait position", "rotate wheel", "sample change complete", "sample rod up", "sample rod down", "retract rod in", "retract rod out", "insert rod in", "insert rod out", "wheel GV open", "wheel GV close", "vent source", "pump source"]
          }
        }
      }
      frame "retract rod in" {
        n161 = Increment(x=w335) -> (x+1=w322:u32)
        n162 = shared-variable "SCA-cRIO\\Mod8\\Retract Rod Actuator"(TRUE ("Sample Rod Actuator")) -> (error out=w326:errorcluster)  [unwired: 1 in]
        n163 = shared-variable ".\\local SCA shared var lib - old.lvlib\\Retract Rod Max Count"() -> (w320:u32)  [unwired: 1 in, 1 out]
        n164 = call "Modify array of SCA states.vi"("Current State"=w328, "Array of states to process"=w329) -> ("Next State"=w330:T7)  [unwired: 7 in, 1 out]
        n165 = shared-variable "SCA-cRIO\\global SCA shared var lib.lvlib\\Retract Rod Status"(error in=w326) -> (w325:T4)  [unwired: 1 out]
        n166 = Greater Or Equal?(x=w322, y=w320) -> (x >= y?=w334:bool)
        n167 = shared-variable ".\\local SCA shared var lib - old.lvlib\\Retract Rod Min Count"() -> (w319:u32)  [unwired: 1 in, 1 out]
        n168 = Equal?(x=w325, y=Horizontal_Rod_states."rod in" ("Enum")) -> (x = y?=w324:bool)
        n169 = Select(t=w342, s=w324, f=u32 0) -> (s? t:f=w340:u32)
        n170 = Increment(x=w340) -> (x+1=w323:u32)
        n171 = Greater Or Equal?(x=w323, y=w319) -> (x >= y?=w341:bool)
        n172 = Select(t=w330, s=w341, f=w328) -> (s? t:f=w337:T7)
        n173 = case shown="True" w334 {
          tunnel: [w348 u32 0] -> w333
          tunnel: [w346 w349] -> w331
          tunnel: [w347 SCA_states."retract rod out" ("SC2 state")] -> w336
          tunnel: w322 -> [w348 _]
          tunnel: w328 -> [w344 _]
          tunnel: [w343 "retract rod failure"] -> w338
          tunnel: w337 -> [w347 _]
          tunnel: w329 -> [w346 _]
          frame False {
            n174 = Format Into String(format string="%s", w344) -> (resulting string=w343:string)  [unwired: 2 in, 1 out]
          }
          frame True {
            w349 = T7[] [enum."retract rod out", enum."insert rod out", enum."wait"] items=["initialize", "wait", "change sample start", "change sample", "check position", "wait position", "rotate wheel", "sample change complete", "sample rod up", "sample rod down", "retract rod in", "retract rod out", "insert rod in", "insert rod out", "wheel GV open", "wheel GV close", "vent source", "pump source"]
          }
        }
      }
      frame "retract rod out" {
        n175 = Increment(x=w369) -> (x+1=w356:u32)
        n176 = shared-variable "SCA-cRIO\\Mod8\\Retract Rod Actuator"(FALSE ("Sample Rod Actuator")) -> (error out=w360:errorcluster)  [unwired: 1 in]
        n177 = call "Modify array of SCA states.vi"("Current State"=w362, "Array of states to process"=w363) -> ("Next State"=w364:T7)  [unwired: 7 in, 1 out]
        n178 = shared-variable ".\\local SCA shared var lib - old.lvlib\\Retract Rod Max Count"() -> (w354:u32)  [unwired: 1 in, 1 out]
        n179 = shared-variable "SCA-cRIO\\global SCA shared var lib.lvlib\\Retract Rod Status"(error in=w360) -> (w359:T4)  [unwired: 1 out]
        n180 = Greater Or Equal?(x=w356, y=w354) -> (x >= y?=w368:bool)
        n181 = shared-variable ".\\local SCA shared var lib - old.lvlib\\Retract Rod Min Count"() -> (w353:u32)  [unwired: 1 in, 1 out]
        n182 = Equal?(x=w359, y=Horizontal_Rod_states."rod out" ("Enum")) -> (x = y?=w358:bool)
        n183 = Select(t=w376, s=w358, f=u32 0) -> (s? t:f=w374:u32)
        n184 = Increment(x=w374) -> (x+1=w357:u32)
        n185 = Greater Or Equal?(x=w357, y=w353) -> (x >= y?=w375:bool)
        n186 = Select(t=w364, s=w375, f=w362) -> (s? t:f=w371:T7)
        n187 = case shown="False" w368 {
          tunnel: [w382 u32 0] -> w367
          tunnel: [w380 w383] -> w365
          tunnel: [w381 SCA_states."retract rod out" ("SC2 state")] -> w370
          tunnel: w356 -> [w382 _]
          tunnel: w362 -> [w378 _]
          tunnel: [w377 "retract rod failure"] -> w372
          tunnel: w371 -> [w381 _]
          tunnel: w363 -> [w380 _]
          frame False {
            n188 = Format Into String(format string="%s", w378) -> (resulting string=w377:string)  [unwired: 2 in, 1 out]
          }
          frame True {
            w383 = T7[] [enum."retract rod out", enum."insert rod out", enum."wait"] items=["initialize", "wait", "change sample start", "change sample", "check position", "wait position", "rotate wheel", "sample change complete", "sample rod up", "sample rod down", "retract rod in", "retract rod out", "insert rod in", "insert rod out", "wheel GV open", "wheel GV close", "vent source", "pump source"]
          }
        }
      }
      frame "insert rod in" {
        n189 = Increment(x=w403) -> (x+1=w390:u32)
        n190 = shared-variable "SCA-cRIO\\Mod8\\Insert Rod Actuator"(TRUE ("Sample Rod Actuator")) -> (error out=w394:errorcluster)  [unwired: 1 in]
        n191 = call "Modify array of SCA states.vi"("Current State"=w396, "Array of states to process"=w397) -> ("Next State"=w398:T7)  [unwired: 7 in, 1 out]
        n192 = shared-variable ".\\local SCA shared var lib - old.lvlib\\Insert Rod Max Count"() -> (w388:u32)  [unwired: 1 in, 1 out]
        n193 = shared-variable "SCA-cRIO\\global SCA shared var lib.lvlib\\Insert Rod Status"(error in=w394) -> (w393:T4)  [unwired: 1 out]
        n194 = Greater Or Equal?(x=w390, y=w388) -> (x >= y?=w402:bool)
        n195 = shared-variable ".\\local SCA shared var lib - old.lvlib\\Insert Rod Min Count"() -> (w387:u32)  [unwired: 1 in, 1 out]
        n196 = Equal?(x=w393, y=Horizontal_Rod_states."rod in" ("Enum")) -> (x = y?=w392:bool)
        n197 = Select(t=w410, s=w392, f=u32 0) -> (s? t:f=w408:u32)
        n198 = Increment(x=w408) -> (x+1=w391:u32)
        n199 = Greater Or Equal?(x=w391, y=w387) -> (x >= y?=w409:bool)
        n200 = Select(t=w398, s=w409, f=w396) -> (s? t:f=w405:T7)
        n201 = case shown="True" w402 {
          tunnel: [w416 u32 0] -> w401
          tunnel: [w414 w417] -> w399
          tunnel: [w415 SCA_states."insert rod out" ("SC2 state")] -> w404
          tunnel: w390 -> [w416 _]
          tunnel: w396 -> [w412 _]
          tunnel: [w411 "insert rod failure"] -> w406
          tunnel: w405 -> [w415 _]
          tunnel: w397 -> [w414 _]
          frame False {
            n202 = Format Into String(format string="%s", w412) -> (resulting string=w411:string)  [unwired: 2 in, 1 out]
          }
          frame True {
            w417 = T7[] [enum."insert rod out", enum."retract rod out", enum."wait"] items=["initialize", "wait", "change sample start", "change sample", "check position", "wait position", "rotate wheel", "sample change complete", "sample rod up", "sample rod down", "retract rod in", "retract rod out", "insert rod in", "insert rod out", "wheel GV open", "wheel GV close", "vent source", "pump source"]
          }
        }
      }
      frame "insert rod out" {
        n203 = Increment(x=w437) -> (x+1=w424:u32)
        n204 = shared-variable ".\\local SCA shared var lib - old.lvlib\\Insert Rod Max Count"() -> (w422:u32)  [unwired: 1 in, 1 out]
        n205 = shared-variable "SCA-cRIO\\Mod8\\Insert Rod Actuator"(FALSE ("Sample Rod Actuator")) -> (error out=w428:errorcluster)  [unwired: 1 in]
        n206 = call "Modify array of SCA states.vi"("Current State"=w430, "Array of states to process"=w431) -> ("Next State"=w432:T7)  [unwired: 7 in, 1 out]
        n207 = shared-variable "SCA-cRIO\\global SCA shared var lib.lvlib\\Insert Rod Status"(error in=w428) -> (w427:T4)  [unwired: 1 out]
        n208 = Greater Or Equal?(x=w424, y=w422) -> (x >= y?=w436:bool)
        n209 = shared-variable ".\\local SCA shared var lib - old.lvlib\\Insert Rod Min Count"() -> (w421:u32)  [unwired: 1 in, 1 out]
        n210 = Equal?(x=w427, y=Horizontal_Rod_states."rod out" ("Enum")) -> (x = y?=w426:bool)
        n211 = Select(t=w444, s=w426, f=u32 0) -> (s? t:f=w442:u32)
        n212 = Increment(x=w442) -> (x+1=w425:u32)
        n213 = Greater Or Equal?(x=w425, y=w421) -> (x >= y?=w443:bool)
        n214 = Select(t=w432, s=w443, f=w430) -> (s? t:f=w439:T7)
        n215 = case shown="False" w436 {
          tunnel: [w450 u32 0] -> w435
          tunnel: [w448 w451] -> w433
          tunnel: [w449 SCA_states."insert rod out" ("SC2 state")] -> w438
          tunnel: w424 -> [w450 _]
          tunnel: w430 -> [w446 _]
          tunnel: [w445 "insert rod failure"] -> w440
          tunnel: w439 -> [w449 _]
          tunnel: w431 -> [w448 _]
          frame False {
            n216 = Format Into String(format string="%s", w446) -> (resulting string=w445:string)  [unwired: 2 in, 1 out]
          }
          frame True {
            w451 = T7[] [enum."insert rod out", enum."retract rod out", enum."wait"] items=["initialize", "wait", "change sample start", "change sample", "check position", "wait position", "rotate wheel", "sample change complete", "sample rod up", "sample rod down", "retract rod in", "retract rod out", "insert rod in", "insert rod out", "wheel GV open", "wheel GV close", "vent source", "pump source"]
          }
        }
      }
      frame "rotate wheel" {
        w480 = 10000.0 ("acceleration")
        # "in motor steps"
        # "The counter logic here (along with \"wait position\") doesn't appear to have a clear purpose.  Doesn't appear that the failure state could ever be acheived as the max timer"
        n217 = shared-variable "SCA-cRIO\\global SCA shared var lib.lvlib\\New Move"() -> (w463:dbl)  [unwired: 1 in, 1 out]
        n218 = Increment(x=w477) -> (x+1=w472:u32)
        n219 = Increment(x=w479) -> (x+1=w462:u32)
        n220 = shared-variable ".\\local SCA shared var lib.lvlib\\Motor Status"(FALSE ("Motor Status")) -> ()  [unwired: 1 in, 1 out]
        n221 = feedback #1() -> (w457:bool)  [unwired: 1 in]
        n222 = xnode "Straight-Line Move"("resource"=w481, "execute"=w457, "position"=w463, "velocity"=w480, "acceleration"=w480, "deceleration"=w480, "accel. jerk"=w480, "smoothing"=w480) -> ("error out"=w460:errorcluster, "done"=w468:bool)  [unwired: 2 in, 4 out]
        "done" <- w468
        "Rotate Wheel error" <- w460
        n223 = shared-variable ".\\local SCA shared var lib - old.lvlib\\Rotate Wheel Min Count"() -> (w456:u32)  [unwired: 1 in, 1 out]
        n224 = shared-variable ".\\local SCA shared var lib.lvlib\\Rotate Wheel error"(w460) -> ()  [unwired: 1 in, 1 out]
        n225 = Not(x=w468) -> (.not. x?=w458:bool)
        n226 = feedback-in #1(w458) -> ()
        n227 = local write "Execute Move"(w458) -> ()
        n228 = shared-variable ".\\local SCA shared var lib - old.lvlib\\Rotate Wheel Max Count"() -> (w455:u32)  [unwired: 1 in, 1 out]
        n229 = Greater Or Equal?(x=w462, y=w456) -> (x >= y?=w473:bool)
        n230 = Select(t=u32 0, s=w473, f=w472) -> (s? t:f=w470:u32)
        n231 = Select(t=SCA_states."wait position" ("SC2 state"), s=w468, f=SCA_states."rotate wheel" ("SC2 state")) -> (s? t:f=w469:T7)
        n232 = Greater Or Equal?(x=w472, y=w455) -> (x >= y?=w478:bool)
        n233 = case shown="True" w478 {
          tunnel: [w482 w487] -> w476
          tunnel: [w486 SCA_states."retract rod out" ("SC2 state")] -> w475
          tunnel: w466 -> [w484 _]
          tunnel: [w483 "rotate failure"] -> w474
          tunnel: w469 -> [w486 _]
          tunnel: w467 -> [w482 _]
          frame False {
            n234 = Format Into String(format string="%s", w484) -> (resulting string=w483:string)  [unwired: 2 in, 1 out]
          }
          frame True {
            w487 = T7[] [enum."retract rod out", enum."insert rod out", enum."wait"] items=["initialize", "wait", "change sample start", "change sample", "check position", "wait position", "rotate wheel", "sample change complete", "sample rod up", "sample rod down", "retract rod in", "retract rod out", "insert rod in", "insert rod out", "wheel GV open", "wheel GV close", "vent source", "pump source"]
          }
        }
      }
      frame "wait position" {
        # "It's still unclear the purpose of \"wait posiiton\" state given the logic withi -- . could probably be replaced by having timing check in \"check position\" state (similar to what is done in the SCB project's state machine"
        n235 = Increment(x=w532) -> (x+1=w533:u32)
        n236 = Increment(x=w530) -> (x+1=w526:u32)
        n237 = shared-variable ".\\local SCA shared var lib - old.lvlib\\Wait Position Min Count"() -> (w516:u32)  [unwired: 1 in, 1 out]
        n238 = shared-variable ".\\local SCA shared var lib - old.lvlib\\Wait Position Max Count"() -> (w531:u32)  [unwired: 1 in, 1 out]
        n239 = Greater Or Equal?(x=w533, y=w516) -> (x >= y?=w527:bool)
        n240 = Greater Or Equal?(x=w526, y=w531) -> (x >= y?=w523:bool)
        n241 = Select(t=u32 0, s=w527, f=w526) -> (s? t:f=w524:u32)
        n242 = case shown="True" w523 {
          tunnel: [w537 w538] -> w529
          tunnel: w521 -> [w535 _]
          tunnel: [w534 "rotate failure"] -> w528
          tunnel: w520 -> [w537 _]
          frame False {
            n243 = Format Into String(format string="%s", w535) -> (resulting string=w534:string)  [unwired: 2 in, 1 out]
          }
          frame True {
            w538 = T7[] [enum."retract rod out", enum."insert rod out", enum."wait"] items=["initialize", "wait", "change sample start", "change sample", "check position", "wait position", "rotate wheel", "sample change complete", "sample rod up", "sample rod down", "retract rod in", "retract rod out", "insert rod in", "insert rod out", "wheel GV open", "wheel GV close", "vent source", "pump source"]
          }
        }
        n244 = Select(t=SCA_states."wait position" ("SC2 state"), s=w523, f=SCA_states."check position" ("SC2 state")) -> (s? t:f=w522:T7)
      }
      frame "check position" {
        # "Move in motor steps"
        n245 = shared-variable "SCA-cRIO\\global SCA shared var lib.lvlib\\Encoder position"() -> (w545:i16)  [unwired: 1 in, 1 out]
        n246 = shared-variable "SCA-cRIO\\global SCA shared var lib.lvlib\\Encoder Offset"() -> (w546:i16)  [unwired: 1 in, 1 out]
        n247 = shared-variable ".\\local SCA shared var lib.lvlib\\New sample"() -> (w542:i8)  [unwired: 1 in, 1 out]
        n248 = call "SCA Sample-Encoder conversion.vi"("Step Window Radius"="Step Window Radius", "Rollover Sample"="Rollover Sample", "Encoder Offset"=w545, "Encoder Position"=w546, "Desired Sample"=w542) -> ("Window limit 1"=w541:i16, "Within Range?"=w554:bool, "Encoder destination"=w552:i16, "Window limit 2"=w540:i16, "New move (encoder steps)"=w557:i16)  [unwired: 2 in]
        "Encoder Destination" <- w552
        "In Range?" <- w554
        "Window Limit 2" <- w540
        "Window Limit 1" <- w541
        n249 = shared-variable "SCA-cRIO\\global SCA shared var lib - old.lvlib\\wheel offset plus"(w541) -> ()  [unwired: 1 in, 1 out]
        n250 = shared-variable "SCA-cRIO\\global SCA shared var lib.lvlib\\Encoder Destination"(w552) -> ()  [unwired: 1 in, 1 out]
        n251 = shared-variable "SCA-cRIO\\global SCA shared var lib - old.lvlib\\wheel offset minus"(w540) -> ()  [unwired: 1 in, 1 out]
        n252 = call "Modify array of SCA states.vi"("Current State"=w551, "Array of states to process"=w550) -> ("Next State"=w549:T7)  [unwired: 7 in, 1 out]
        n253 = Select(t=w549, s=w554, f=SCA_states."rotate wheel" ("SC2 state")) -> (s? t:f=w561:T7)
        n254 = shared-variable ".\\local SCA shared var lib.lvlib\\Motor Status"(w554) -> ()  [unwired: 1 in, 1 out]
        n255 = Multiply(x=w557, y=3.0519) -> (x*y=w553:dbl)
        "New Move" <- w553
        n256 = shared-variable "SCA-cRIO\\global SCA shared var lib.lvlib\\New Move"(w553) -> ()  [unwired: 1 in, 1 out]
        n257 = Format Into String(format string="%s", w551) -> (resulting string=w560:string)  [unwired: 2 in, 1 out]
      }
    }
    "action" <- w140
    "SCA next state" <- w144
    n258 = shared-variable "SCA-cRIO\\global SCA shared var lib.lvlib\\Current State"(w134) -> ()  [unwired: 1 in, 1 out]
    n259 = call "Wait Until Next Multiple"("Count(mSec)"=u32 5) -> ()  [unwired: 1 out]
    n260 = shared-variable "SCA-cRIO\\global SCA shared var lib.lvlib\\SC SM counter"(w136) -> ()  [unwired: 1 in, 1 out]
  }
  n261 = while {
    stop <- FALSE stop-if-true
    # "Error reporting - loop reports errors to/from RT/SVE. \nNo RT error: 0.5 Hz blinking\nRT error: 5 Hz blinking"
    n262 = shared-variable ".\\local SCA shared var lib.lvlib\\Convectron readback loop error"() -> (w564:errorcluster)  [unwired: 1 in, 1 out]
    n263 = shared-variable ".\\local SCA shared var lib.lvlib\\Timeouts Update loop error"() -> (w562:errorcluster)  [unwired: 1 in, 1 out]
    n264 = shared-variable ".\\local SCA shared var lib.lvlib\\Vac Readback Loop error"() -> (w569:errorcluster)  [unwired: 1 in, 1 out]
    n265 = shared-variable ".\\local SCA shared var lib.lvlib\\HV Control loop error"() -> (w565:errorcluster)  [unwired: 1 in, 1 out]
    n266 = shared-variable ".\\local SCA shared var lib.lvlib\\Rotate Wheel error"() -> (w566:errorcluster)  [unwired: 1 in, 1 out]
    n267 = shared-variable ".\\local SCA shared var lib.lvlib\\Encoder loop error"() -> (w563:errorcluster)  [unwired: 1 in, 1 out]
    n268 = shared-variable ".\\local SCA shared var lib.lvlib\\Sensor Loop error"() -> (w570:errorcluster)  [unwired: 1 in, 1 out]
    n269 = Merge Errors(w570, w569, w566, w565, w564, w563, w562) -> (w568:errorcluster)
    "SCA-cRIO error" <- w568
    n270 = shared-variable "SCA-cRIO\\global SCA shared var lib.lvlib\\SCA-RT error"(w568) -> ()  [unwired: 1 in, 1 out]
    n271 = case shown="Error" w568 {
      tunnel: 0 -> [w574 w582]
      frame No Error {
        n272 = flat-sequence {
          tunnel: w574 -> [w575]
          tunnel: [w575] -> w572
          tunnel: [w577] -> w573
          tunnel: w572 -> [w577]
          tunnel: w573 -> [w579]
          frame #0 {
            n273 = call <vilib>:"RT LEDs.vi"("State"=3, "LED Num"=w575) -> ()  [unwired: 4 in, 2 out]
          }
          frame #1 {
            n274 = call "Wait"("Count(mSec)"=u16 1000) -> ()  [unwired: 1 out]
          }
          frame #2 {
            n275 = call <vilib>:"RT LEDs.vi"("State"=3, "LED Num"=w579) -> ()  [unwired: 4 in, 2 out]
          }
          frame #3 {
            n276 = call "Wait2"("Count(mSec)"=u16 1000) -> ()  [unwired: 1 out]
          }
        }
      }
      frame Error {
        n277 = flat-sequence {
          tunnel: [w585] -> w584
          tunnel: w582 -> [w585]
          tunnel: w584 -> [w587]
          tunnel: [w587] -> w583
          tunnel: w583 -> [w589]
          frame #0 {
            n278 = call <vilib>:"RT LEDs.vi"("State"=3, "LED Num"=w585) -> ()  [unwired: 4 in, 2 out]
          }
          frame #1 {
            n279 = call "Wait3"("Count(mSec)"=u16 100) -> ()  [unwired: 1 out]
          }
          frame #2 {
            n280 = call <vilib>:"RT LEDs.vi"("State"=3, "LED Num"=w589) -> ()  [unwired: 4 in, 2 out]
          }
          frame #3 {
            n281 = call "Wait4"("Count(mSec)"=u16 100) -> ()  [unwired: 1 out]
          }
        }
      }
    }
  }
  n282 = while {
    shift-right: [w596] -> _
    shift-left: timestamp(0 s since 1904-01-01) -> [w595]
    stop <- FALSE stop-if-true
    # "SCA command monitor -- when timestamp updated, new command processed"
    n283 = shared-variable "SCA-cRIO\\global SCA shared var lib.lvlib\\SCA Command"() -> (w592:T1, w597:timestamp)  [unwired: 1 in, 1 out]
    "SCA Command" <- w592
    n284 = Wait Until Next ms Multiple(millisecond multiple=u32 50) -> ()  [unwired: 1 out]
    n285 = Equal?(x=w597, y=w595) -> (x = y?=w598:bool)
    n286 = case shown="False" w598 {
      tunnel: w597 -> [w601 _]
      tunnel: [w601 w642] -> w596
      tunnel: w595 -> [_ w642]
      tunnel: w592 -> [w600 _]
      frame False {
        n287 = case shown="\"Rotate wheel\"" w600 {
          tunnel: [SCA_states."insert rod out" ("SC2 state") SCA_states."insert rod in" ("SC2 state") SCA_states."retract rod out" ("SC2 state") SCA_states."retract rod in" ("SC2 state") SCA_states."sample rod up" ("SC2 state") SCA_states."sample rod down" ("SC2 state") SCA_states."wheel GV open" ("SC2 state") SCA_states."wheel GV close" ("SC2 state") SCA_states."wait" ("SC2 state") SCA_states."wait" ("SC2 state") SCA_states."pump source" ("SC2 state") SCA_states."vent source" ("SC2 state") w615 w620 w629 w633] -> w599
          frame "Retract insert rod", Default {
          }
          frame "Insert insert rod" {
          }
          frame "Retract retract rod" {
          }
          frame "Insert retract rod" {
          }
          frame "Retract sample rod" {
          }
          frame "Insert sample rod" {
          }
          frame "Open wheel GV" {
          }
          frame "Close wheel GV" {
          }
          frame "Open ion source GV" {
          }
          frame "Close ion source GV" {
          }
          frame "Pump out source" {
          }
          frame "Vent source" {
          }
          frame "Rotate wheel" {
            n288 = shared-variable ".\\local SCA shared var lib.lvlib\\Motor Status"() -> (w614:bool)  [unwired: 1 in, 1 out]
            n289 = case shown="True" w614 {
              tunnel: [SCA_states."wait" ("SC2 state") SCA_states."rotate wheel" ("SC2 state")] -> w615
              frame False {
              }
              frame True {
                n290 = shared-variable "SCA-cRIO\\global SCA shared var lib.lvlib\\Requested Sample"() -> (w617:u8)  [unwired: 1 in, 1 out]
                n291 = shared-variable ".\\local SCA shared var lib.lvlib\\New sample"(w617) -> ()  [unwired: 1 in, 1 out]
              }
            }
          }
          frame "Rotate wheel randomly" {
            n292 = shared-variable ".\\local SCA shared var lib.lvlib\\Motor Status"() -> (w619:bool)  [unwired: 1 in, 1 out]
            n293 = case shown="True" w619 {
              tunnel: [SCA_states."wait" ("SC2 state") SCA_states."rotate wheel" ("SC2 state")] -> w620
              frame False {
              }
              frame True {
                n294 = Random Number (0-1)() -> (number: 0 to 1=w625:dbl)
                n295 = Multiply(x=w625, y=63.0) -> (x*y=w623:dbl)
                n296 = Round Toward +Infinity(x=w623) -> (ceil(x): smallest int >= x=w626:dbl)
                n297 = To Unsigned Byte Integer(number=w626) -> (unsigned 8bit integer=w622:u8)
                n298 = shared-variable ".\\local SCA shared var lib.lvlib\\New sample"(w622) -> ()  [unwired: 1 in, 1 out]
              }
            }
          }
          frame "Start sample change" {
            n299 = shared-variable ".\\local SCA shared var lib.lvlib\\Motor Status"() -> (w628:bool)  [unwired: 1 in, 1 out]
            n300 = case shown="False" w628 {
              tunnel: [SCA_states."wait" ("SC2 state") SCA_states."change sample" ("SC2 state")] -> w629
              frame False {
              }
              frame True {
                n301 = shared-variable "SCA-cRIO\\global SCA shared var lib.lvlib\\Requested Sample"() -> (w631:u8)  [unwired: 1 in, 1 out]
                n302 = shared-variable ".\\local SCA shared var lib.lvlib\\New sample"(w631) -> ()  [unwired: 1 in, 1 out]
              }
            }
          }
          frame "Start random sample change" {
            n303 = shared-variable ".\\local SCA shared var lib.lvlib\\Motor Status"() -> (w634:bool)  [unwired: 1 in, 1 out]
            n304 = case shown="True" w634 {
              tunnel: [SCA_states."wait" ("SC2 state") SCA_states."change sample" ("SC2 state")] -> w633
              frame False {
              }
              frame True {
                n305 = Random Number (0-1)() -> (number: 0 to 1=w639:dbl)
                n306 = Multiply(x=w639, y=63.0) -> (x*y=w637:dbl)
                n307 = Round Toward +Infinity(x=w637) -> (ceil(x): smallest int >= x=w640:dbl)
                n308 = To Unsigned Byte Integer(number=w640) -> (unsigned 8bit integer=w636:u8)
                n309 = shared-variable ".\\local SCA shared var lib.lvlib\\New sample"(w636) -> ()  [unwired: 1 in, 1 out]
              }
            }
          }
        }
        n310 = shared-variable ".\\local SCA shared var lib.lvlib\\SCA state control"(w599) -> ()  [unwired: 1 in, 1 out]
      }
      frame True {
      }
    }
  }
  n311 = node-c288() -> (w6:T9)  [unwired: 4 in]
  n312 = while {
    shift-right: [w659] -> _
    shift-left: 0.0 ("AI1") -> [w662]
    shift-right: [w657] -> _
    shift-left: w3 -> [w656]
    shift-right: [w658] -> _
    shift-left: w3 -> [w655]
    shift-right: [w653] -> _
    shift-left: w3 -> [w652]
    shift-right: [w650] -> _
    shift-left: w3 -> [w649]
    shift-right: [w644] -> _
    shift-left: w3 -> [w647]
    shift-right: [w643] -> _
    shift-left: w3 -> [w648]
    stop <- FALSE stop-if-true
    # "HV readback loop"
    n313 = shared-variable "SCA-cRIO\\Mod5\\Immersion Lens V read"() -> (w645:dbl)  [unwired: 1 in, 1 out]
    n314 = shared-variable "SCA-cRIO\\Mod5\\Immersion Lens I read"() -> (w646:dbl)  [unwired: 1 in, 1 out]
    n315 = Wait Until Next ms Multiple(millisecond multiple=u32 10) -> ()  [unwired: 1 out]
    n316 = Greater Or Equal?(x=w662, y=100.0) -> (x >= y?=w660:bool)
    n317 = shared-variable "SCA-cRIO\\Mod5\\Extractor V read"() -> (w654:dbl)  [unwired: 1 in, 1 out]
    n318 = shared-variable "SCA-cRIO\\Mod5\\Extractor I read"() -> (w651:dbl)  [unwired: 1 in, 1 out]
    n319 = shared-variable "SCA-cRIO\\Mod5\\Cathode V read"() -> (w664:dbl)  [unwired: 1 in, 1 out]
    n320 = shared-variable "SCA-cRIO\\Mod5\\Cathode I read"() -> (w663:dbl)  [unwired: 1 in, 1 out]
    n321 = case shown="True" w660 {
      tunnel: w664 -> [w682 _]
      tunnel: w663 -> [w683 _]
      tunnel: w662 -> [w686 _]
      tunnel: [w685 0.0 ("AI1")] -> w659
      tunnel: [w684 w690] -> w658
      tunnel: [w681 w690] -> w657
      tunnel: w656 -> [w680 w698]
      tunnel: w655 -> [w679 w699]
      tunnel: w654 -> [w678 _]
      tunnel: [w677 w690] -> w653
      tunnel: w652 -> [w676 w697]
      tunnel: w651 -> [w675 _]
      tunnel: [w674 w690] -> w650
      tunnel: w649 -> [w673 w696]
      tunnel: w648 -> [w672 w689]
      tunnel: w647 -> [w671 w688]
      tunnel: w646 -> [w670 _]
      tunnel: w645 -> [w669 _]
      tunnel: [w668 w690] -> w644
      tunnel: [w667 w690] -> w643
      frame False {
        n322 = Build Array (concatenate)(w670, w671) -> (w668:dbl[])
        n323 = Build Array (concatenate)(w669, w672) -> (w667:dbl[])
        n324 = Build Array (concatenate)(w683, w679) -> (w684:dbl[])
        n325 = Build Array (concatenate)(w682, w680) -> (w681:dbl[])
        n326 = Build Array (concatenate)(w678, w676) -> (w677:dbl[])
        n327 = Build Array (concatenate)(w675, w673) -> (w674:dbl[])
        n328 = Increment(x=w686) -> (x+1=w685:dbl)
      }
      frame True {
        w690 = dbl[] []
        n329 = call-poly <vilib>:"Mean.vi"("X"=w688) -> ("mean"=w687:dbl)  [unwired: 1 out]
        "Immersion Lens I read" <- w687
        n330 = call-poly <vilib>:"Mean.vi"("X"=w689) -> ("mean"=w691:dbl)  [unwired: 1 out]
        "Immersion Lens V read" <- w691
        n331 = call-poly <vilib>:"Mean.vi"("X"=w699) -> ("mean"=w695:dbl)  [unwired: 1 out]
        "Cathode I read" <- w695
        n332 = call-poly <vilib>:"Mean.vi"("X"=w698) -> ("mean"=w694:dbl)  [unwired: 1 out]
        "Cathode V read" <- w694
        n333 = call-poly <vilib>:"Mean.vi"("X"=w697) -> ("mean"=w693:dbl)  [unwired: 1 out]
        "Extractor V read" <- w693
        n334 = call-poly <vilib>:"Mean.vi"("X"=w696) -> ("mean"=w692:dbl)  [unwired: 1 out]
        "Extractor I read" <- w692
        n335 = shared-variable "SCA-cRIO\\global SCA shared var lib.lvlib\\Immersion Lens I read"(w687) -> ()  [unwired: 1 in, 1 out]
        n336 = shared-variable "SCA-cRIO\\global SCA shared var lib.lvlib\\Immersion Lens V read"(w691) -> ()  [unwired: 1 in, 1 out]
        n337 = shared-variable "SCA-cRIO\\global SCA shared var lib.lvlib\\Cathode I read"(w695) -> ()  [unwired: 1 in, 1 out]
        n338 = shared-variable "SCA-cRIO\\global SCA shared var lib.lvlib\\Cathode V read"(w694) -> ()  [unwired: 1 in, 1 out]
        n339 = shared-variable "SCA-cRIO\\global SCA shared var lib.lvlib\\Extractor V read"(w693) -> ()  [unwired: 1 in, 1 out]
        n340 = shared-variable "SCA-cRIO\\global SCA shared var lib.lvlib\\Extractor I read"(w692) -> ()  [unwired: 1 in, 1 out]
      }
    }
  }
  n341 = timed-loop {
    timing: w6 -> [_]
    timing-out: [_] -> w5
    stop <- FALSE stop-if-true
    # "Encoder readback loop"
    n342 = node-c288() -> ()  [unwired: 1 in, 1 out]
    n343 = shared-variable "SCA-cRIO\\Mod6\\DIO0"() -> (w733:bool, error out=w716:errorcluster)  [unwired: 1 in]
    n344 = shared-variable "SCA-cRIO\\Mod6\\DIO1"(error in=w716) -> (w732:bool, error out=w715:errorcluster)
    n345 = shared-variable "SCA-cRIO\\Mod6\\DIO2"(error in=w715) -> (w723:bool, error out=w714:errorcluster)
    n346 = shared-variable "SCA-cRIO\\Mod6\\DIO3"(error in=w714) -> (w722:bool, error out=w713:errorcluster)
    n347 = shared-variable "SCA-cRIO\\Mod6\\DIO4"(error in=w713) -> (w731:bool, error out=w712:errorcluster)
    n348 = shared-variable "SCA-cRIO\\Mod6\\DIO5"(error in=w712) -> (w730:bool, error out=w711:errorcluster)
    n349 = shared-variable "SCA-cRIO\\Mod6\\DIO6"(error in=w711) -> (w729:bool, error out=w710:errorcluster)
    n350 = shared-variable "SCA-cRIO\\Mod6\\DIO7"(error in=w710) -> (w709:bool, error out=w708:errorcluster)
    n351 = shared-variable "SCA-cRIO\\Mod6\\DIO8"(error in=w708) -> (w728:bool, error out=w707:errorcluster)
    n352 = shared-variable "SCA-cRIO\\Mod6\\DIO9"(error in=w707) -> (w721:bool, error out=w706:errorcluster)
    n353 = shared-variable "SCA-cRIO\\Mod6\\DIO10"(error in=w706) -> (w727:bool, error out=w705:errorcluster)
    n354 = shared-variable "SCA-cRIO\\Mod6\\DIO11"(error in=w705) -> (w726:bool, error out=w704:errorcluster)
    n355 = shared-variable "SCA-cRIO\\Mod6\\DIO12"(error in=w704) -> (w725:bool, error out=w703:errorcluster)
    n356 = shared-variable "SCA-cRIO\\Mod6\\DIO13"(error in=w703) -> (w724:bool, error out=w702:errorcluster)
    n357 = Bundle By Name(cluster=T12 {"MSB"=FALSE, "13th bit"=FALSE, "12th bit"=FALSE, "11th bit"=FALSE, "10th bit"=FALSE, "9th bit"=FALSE, "8th bit"=FALSE, "7th bit"=FALSE, "6th bit"=FALSE, "5th bit"=FALSE, "4th bit"=FALSE, "3rd bit"=FALSE, "2nd bit"=FALSE, "LSB"=FALSE} ("Cluster"), "MSB"=w733, "13th bit"=w732, "12th bit"=w723, "11th bit"=w722, "10th bit"=w731, "9th bit"=w730, "8th bit"=w729, "7th bit"=w709, "6th bit"=w728, "5th bit"=w721, "4th bit"=w727, "3rd bit"=w726, "2nd bit"=w725, "LSB"=w724) -> (w735:T12)
    n358 = call "Encoder-Decoder.vi"("Encoder data"=w735) -> ("Raw bits"=→"Raw bits":bool[], "Converted bits"=→"Converted bits":bool[], "Encoder position"=w720:u16)  [unwired: 8 in]
    "Encoder position" <- w720
    n359 = shared-variable "SCA-cRIO\\global SCA shared var lib.lvlib\\Encoder position"(w720, error in=w702) -> (error out=w701:errorcluster)
    "Encoder loop error" <- w701
    n360 = shared-variable ".\\local SCA shared var lib.lvlib\\Encoder loop error"(w701) -> ()  [unwired: 1 in, 1 out]
    n361 = node-c288() -> ()  [unwired: 1 in, 1 out]
  }
  n362 = node-c288(w5) -> ()  [unwired: 1 out]
